vi "Constructor.vi"(8 "error in (no error)":errorcluster, 11 "FreshClams in":refnum<class "FreshClams.lvclass">) -> (0 "error out":errorcluster, 2 "Ingredients":string, 3 "FreshClams out":refnum<class "FreshClams.lvclass">)   [LabVIEW 2013, in "FreshClams.lvclass"]
uses:
  FreshClams.lvclass
panel:
  # "§Ú¬O·sÂA¥Íµð¸Ä"
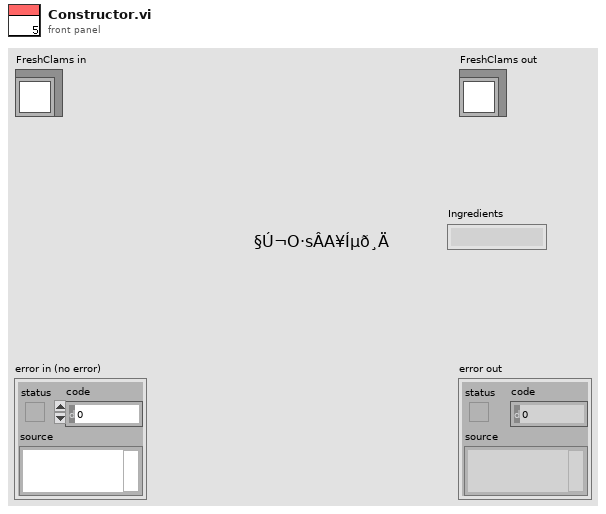
[diagram p1: front panel]
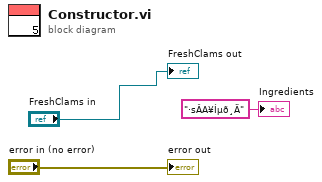
[diagram p0: block diagram]
diagram:
  "error out" <- "error in (no error)"
  "FreshClams out" <- "FreshClams in"
  "Ingredients" <- "·sÂA¥Íµð¸Ä" ("Ingredients")
